vi "取中心点.vi"(10 "前面板窗口:最小尺寸":T1 caption="点", 11 "显示:主工作区":T2) -> (3 "前面板窗口:窗口边界":T2 caption="矩形")   [LabVIEW 2016, in "斯坦道总磷.lvlib"]
uses:
  <vilib>/Utility/miscctls.llb/LVRectTypeDef.ctl
  <vilib>/Utility/miscctls.llb/LVPointTypeDef.ctl
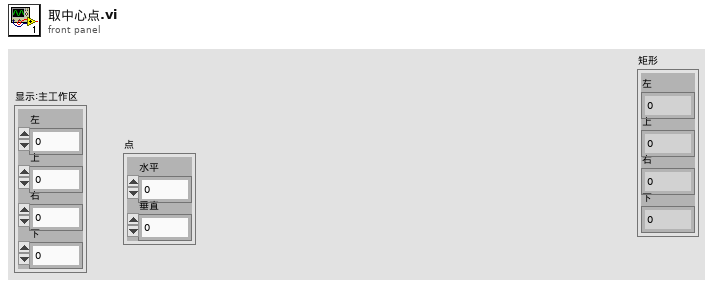
[diagram p1: front panel]
types:
  T1 = typedef "LVPointTypeDef.ctl" = cluster{"Horizontal":i16, "Vertical":i16}
  T2 = typedef "LVRectTypeDef.ctl" = cluster{"Left":i16, "Top":i16, "Right":i16, "Bottom":i16}
  T3 = cluster{"Left":sgl, "Top":sgl, "Right":sgl, "Bottom":sgl}
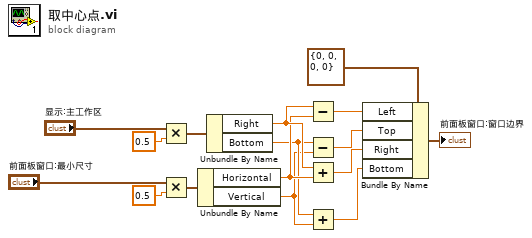
[diagram p0: block diagram]
diagram:
  n1 = Multiply(x="显示:主工作区", y=sgl 0.5) -> (x*y=w11:T3)
  n2 = Multiply(x="前面板窗口:最小尺寸", y=sgl 0.5) -> (x*y=w10:cluster{"Horizontal":sgl, "Vertical":sgl})
  n3 = Unbundle By Name(w10) -> ("Horizontal"=w6:sgl, "Vertical"=w3:sgl)
  n4 = Unbundle By Name(w11) -> ("Right"=w7:sgl, "Bottom"=w4:sgl)
  n5 = Subtract(x=w7, y=w6) -> (x-y=w9:sgl)
  n6 = Subtract(x=w4, y=w3) -> (x-y=w8:sgl)
  n7 = Add(x=w7, y=w6) -> (x+y=w5:sgl)
  n8 = Add(x=w4, y=w3) -> (x+y=w2:sgl)
  n9 = Bundle By Name(cluster=T2 {"Left"=0, "Top"=0, "Right"=0, "Bottom"=0} ("前面板窗口:窗口边界"), "Left"=w9, "Top"=w8, "Right"=w5, "Bottom"=w2) -> (→"前面板窗口:窗口边界":T2)
